vi "Autonomous Independent.vi"() -> ()   [LabVIEW 2016]
doc: "This VI is called when autonomous begins, and will automatically be terminated when autonomous ends. You can carry out timed or sensor driven robot movement independently without needing to return to the caller."
uses:
  <vilib>/Rock Robotics/WPI/DriverStation/WPI_DriverStationAllianceInfo.ctl
  Controls/Auto Selector.ctl
  Controls/Auto 1.ctl
  Controls/Auto 2.ctl
  Controls/Control 1.ctl
  Robot Global Data.vi
  <vilib>/Rock Robotics/Network Tables/NT Read Number.vi
panel:
  in  "4th distance C":dbl=2.0 format="%#_13g"
  in  "2nd Turn":dbl=49.0
  in  "3rd distance C":dbl=-0.5
  in  "2nd distance C":dbl=0.6 format="%#_13g"
  in  "1st turn C":dbl=-49.0
  in  "1st distance C":dbl=1.7
  in  "Turret angle Blue":dbl=13.0
  in  "CORRECAO":dbl=0.02
  in  "2nd distance B":dbl=0.3 format="%#_13g"
  in  "1st distance B":dbl=1.5 format="%#_13g"
  out "Red alliance?":bool
  in  "Turret angle Red":dbl=-12.0
  in  "3rd distance":dbl=-0.3 format="%#_13g"
  in  "2nd distance":dbl=0.6 format="%#_13g"
  in  "1st turn":dbl=-49.0 format="%.2f"
  in  "1st distance":dbl=1.7 format="%#_13g"
  # "vermelho = -12"
  # "azul = -13"
  # "Gear + Fuel"
  # "Gear on Feeder peg"
  # "Middle Gear"
  # "da pra reduzir  a velocidade segunda distancia"
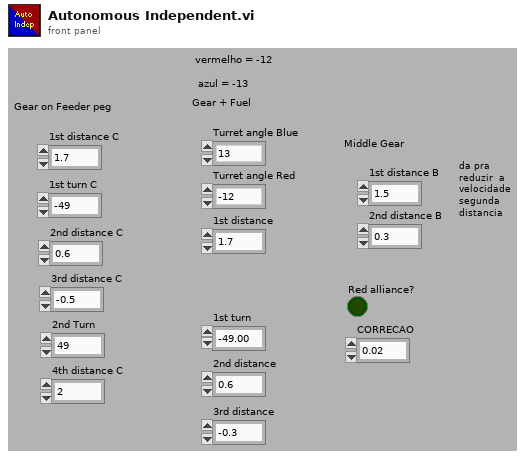
[diagram p1: front panel]
types:
  T1 = typedef "WPI_DriverStationAllianceInfo.ctl" = enum16{"Red", "Blue", "Invalid"}
  T2 = typedef "WPI_EncoderDevRef.ctl" = cluster{"DevStatus":errorcluster, "EncoderIndex":T3, "CounterIndex":T4, "DistancePerCount":dbl, "Decoding Type":T5}
  T3 = typedef "FPGA_EncoderIdx.ctl" = enum8{"Enc 0", "Enc 1", "Enc 2", "Enc 3", "Enc 4", "Enc 5", "Enc 6", "Enc 7", "Invalid"}
  T4 = typedef "FPGA_CounterCtrSystemIndex.ctl" = enum8{"Ctr 0", "Ctr 1", "Ctr 2", "Ctr 3", "Ctr 4", "Ctr 5", "Ctr 6", "Ctr 7", "Invalid"}
  T5 = typedef "WPI_EncoderType.ctl" = enum16{"1x", "2x", "4x"}
  T6 = cluster{"Yaw":dbl, "Roll":dbl, "Pitch":dbl, "Heading":dbl, "Fused Heading":dbl}
  T7 = typedef "Auto Selector.ctl" = enum16{"Gear + Fuel with Vision", "Gear + Fuel no Vision", "Middle Gear", "Gear - Feeder peg", "Nothing"}
  T8 = typedef "Auto 1.ctl" = enum16{"Prepare", "Go Forward 1", "Wait 1", "Turn Left", "Wait 2", "Go Forward 2", "Open Gear Manipulator", "Go Back", "Wait 3"}
  T9 = typedef "Auto 2.ctl" = enum16{"Prepare", "Forward", "Open", "Go Back"}
  T10 = typedef "Control 1.ctl" = enum16{"Prepare", "Go Forward 1", "Wait 1", "Turn 1", "Wait 2", "Go Forward 2", "Drop Gear", "Wait 3", "Go Back", "Wait 4", "Turn 2", "Go forward"}
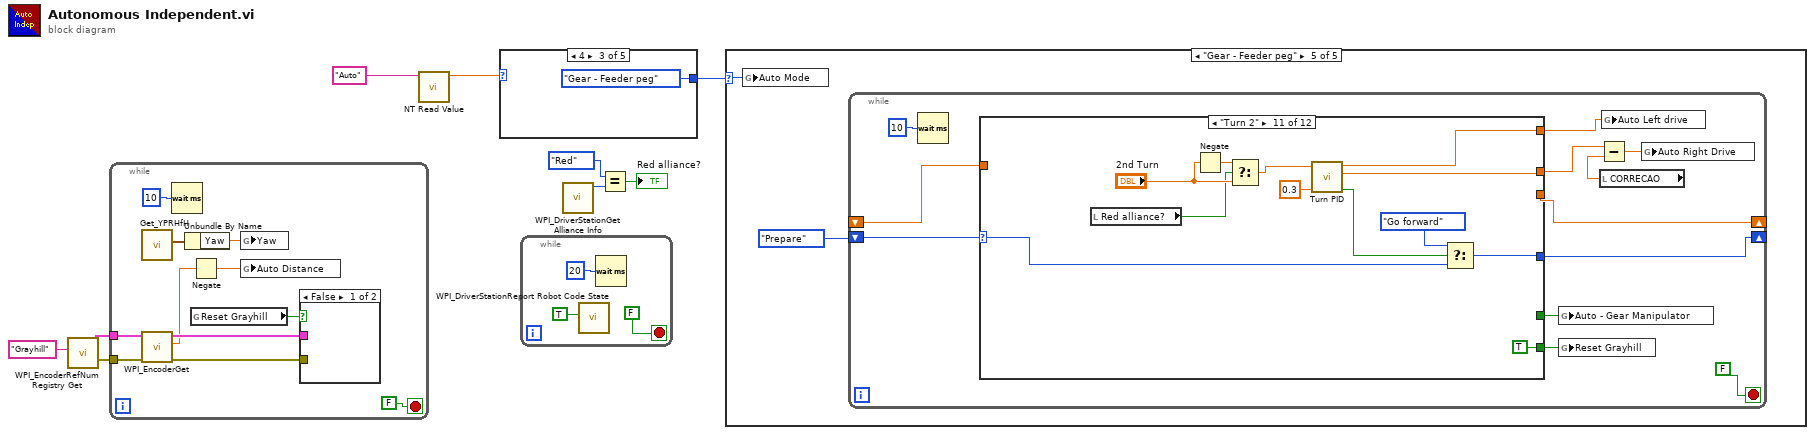
[diagram p0: block diagram]
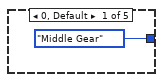
[diagram p2: hidden frame]
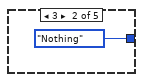
[diagram p3: hidden frame]
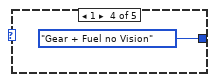
[diagram p4: hidden frame]
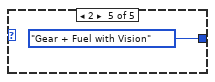
[diagram p5: hidden frame]
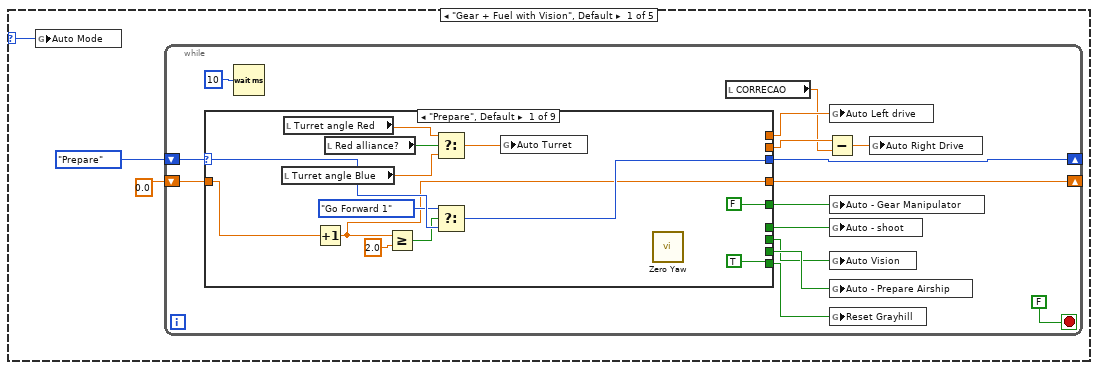
[diagram p6: hidden frame]
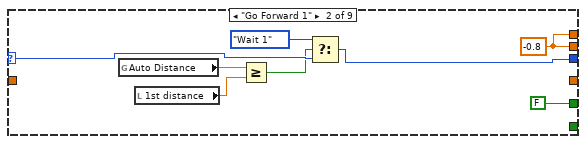
[diagram p7: hidden frame]
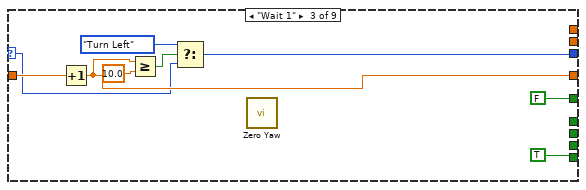
[diagram p8: hidden frame]
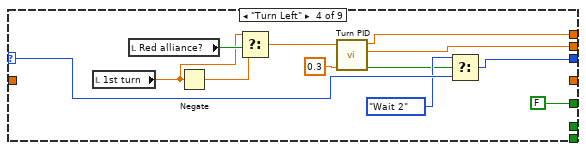
[diagram p9: hidden frame]
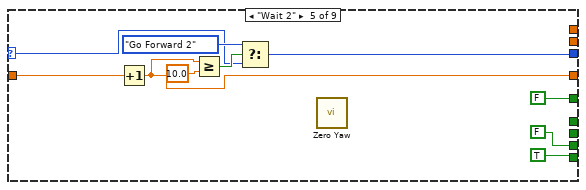
[diagram p10: hidden frame]
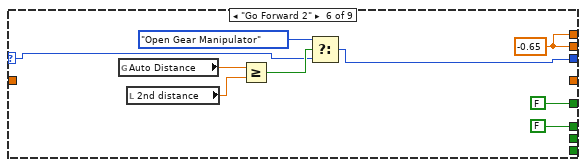
[diagram p11: hidden frame]
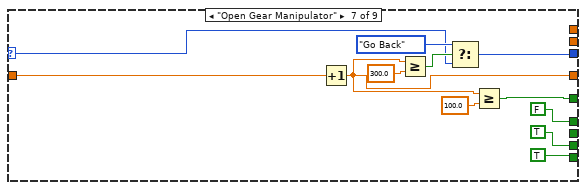
[diagram p12: hidden frame]
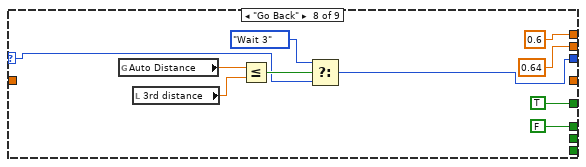
[diagram p13: hidden frame]
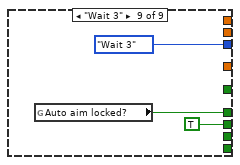
[diagram p14: hidden frame]
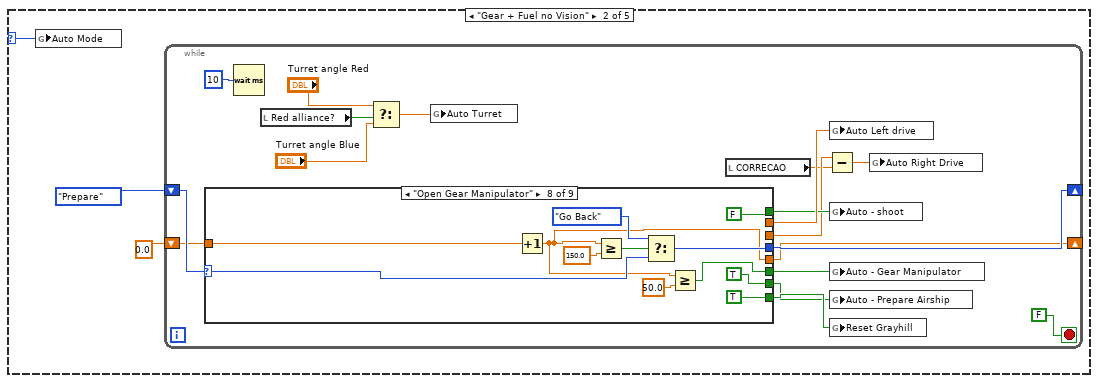
[diagram p15: hidden frame]
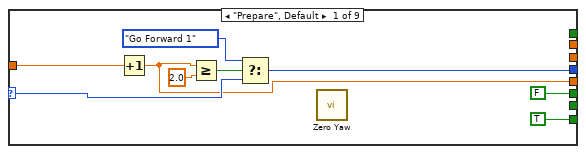
[diagram p16: hidden frame]
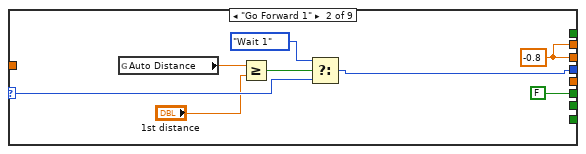
[diagram p17: hidden frame]
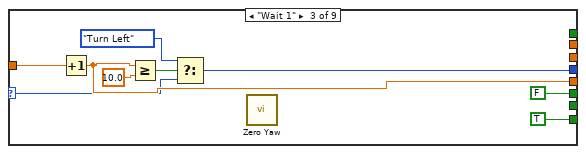
[diagram p18: hidden frame]
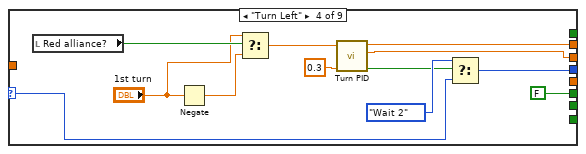
[diagram p19: hidden frame]
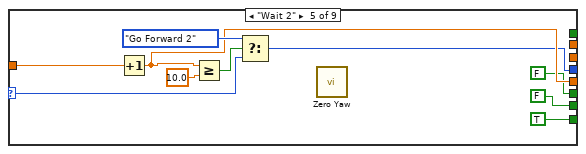
[diagram p20: hidden frame]
diagram:
  n1 = call <vilib>:"WPI_EncoderRefNum Registry Get.vi"("refnum name"="Grayhill") -> ("error out"=w7:errorcluster, "EncoderDevRef"=w8:T2)  [unwired: 9 in]
  n2 = while {
    tunnel: w8 -> [w20]
    tunnel: w7 -> [w19]
    stop <- FALSE stop-if-true
    n3 = call <vilib>:"Get_YPRHfH.vi"() -> ("YRPHfH"=w13:T6)  [unwired: 11 in]
    n4 = call <vilib>:"WPI_EncoderGet.vi"("error in (no error)"=w19, "EncoderDevRef"=w20) -> ("error out"=w17:errorcluster, "Distance"=w11:dbl, "EncoderDevRef"=w18:T2)  [unwired: 4 in, 3 out]
    n5 = Wait (ms)(milliseconds to wait=u32 10) -> ()  [unwired: 1 out]
    n6 = Unbundle By Name(w13) -> ("Yaw"=w12:dbl)
    n7 = Negate(x=w11) -> (-x=w10:dbl)
    n8 = global read "Robot Global Data.vi" "Reset Grayhill"() -> (w16:bool)
    n9 = global write "Robot Global Data.vi" "Yaw"(w12) -> ()
    n10 = global write "Robot Global Data.vi" "Auto Distance"(w10) -> ()
    n11 = case shown="False" w16 {
      tunnel: w18 -> [_ w22]
      tunnel: w17 -> [_ w21]
      frame False {
      }
      frame True {
        n12 = call <vilib>:"WPI_EncoderReset.vi"("error in (no error)"=w21, "EncoderDevRef"=w22) -> ()  [unwired: 8 in, 2 out]
      }
    }
  }
  n13 = call-poly <vilib>:"NT Read Value.vi"("Name"="Auto") -> ("Numeric"=w1:dbl)  [unwired: 9 in, 1 out]
  n14 = case shown="4" w1 {
    tunnel: [Auto_Selector."Middle Gear" Auto_Selector."Nothing" Auto_Selector."Gear - Feeder peg" Auto_Selector."Gear + Fuel no Vision" Auto_Selector."Gear + Fuel with Vision"] -> w3
    frame 0, Default {
    }
    frame 3 {
    }
    frame 4 {
    }
    frame 1 {
    }
    frame 2 {
    }
  }
  n15 = while {
    stop <- FALSE stop-if-true
    n16 = call <vilib>:"WPI_DriverStationReport Robot Code State.vi"("Autonomous"=TRUE) -> ()  [unwired: 10 in, 1 out]
    n17 = Wait (ms)(milliseconds to wait=u32 20) -> ()  [unwired: 1 out]
  }
  n18 = call <vilib>:"WPI_DriverStationGet Alliance Info.vi"() -> ("Alliance"=w6:T1)  [unwired: 11 out]
  n19 = Equal?(x=WPI_DriverStationAllianceInfo."Red" ("Alliance"), y=w6) -> (x = y?=→"Red alliance?":bool)
  n20 = case shown="\"Gear - Feeder peg\"" w3 {
    selector: w3 -> [w31 w135 w237 _ w286]
    frame "Gear + Fuel with Vision", Default {
      n21 = global write "Robot Global Data.vi" "Auto Mode"(w31) -> ()
      n22 = while {
        shift-right: [w46] -> _
        shift-left: Auto_1."Prepare" -> [w47]
        shift-right: [w44] -> _
        shift-left: 0.0 -> [w45]
        stop <- FALSE stop-if-true
        n23 = case shown="\"Prepare\", Default" w47 {
          selector: w47 -> [w60 w67 w74 w86 w94 w106 w115 w126 _]
          tunnel: [w61 w68 w75 w87 w95 w105 w118 w127 Auto_1."Wait 3"] -> w46
          tunnel: w45 -> [w58 _ w78 _ w97 _ w119 _ _]
          tunnel: [w57 _ w77 _ w96 _ w113 _ _] -> w44
          tunnel: [TRUE ("Reset Grayhill") _ TRUE ("Reset Grayhill") _ TRUE ("Reset Grayhill") _ TRUE ("Reset Grayhill") _ _] -> w42
          tunnel: [_ w69 _ w89 _ w104 _ 0.64 ("Right Out") _] -> w36
          tunnel: [_ w69 _ w88 _ w104 _ 0.6 _] -> w41
          tunnel: [FALSE ("Reset Grayhill") FALSE ("Reset Grayhill") FALSE ("Reset Grayhill") FALSE ("Reset Grayhill") FALSE ("Reset Grayhill") FALSE ("Reset Grayhill") w111 TRUE ("Reset Grayhill") _] -> w40
          tunnel: [_ _ _ _ _ FALSE FALSE FALSE w132] -> w39
          tunnel: [_ _ _ _ FALSE ("Reset Grayhill") _ TRUE ("Reset Grayhill") _ _] -> w38
          tunnel: [_ _ _ _ _ _ _ _ TRUE] -> w37
          frame "Prepare", Default {
            n24 = local read "Turret angle Blue"() -> (w49:dbl)
            n25 = local read "Turret angle Red"() -> (w50:dbl)
            n26 = Increment(x=w58) -> (x+1=w57:dbl)
            n27 = local read "Red alliance?"() -> (w51:bool)
            n28 = Greater Or Equal?(x=w57, y=2.0) -> (x >= y?=w55:bool)
            n29 = Select(t=w50, s=w51, f=w49) -> (s? t:f=w52:dbl)
            n30 = Select(t=Auto_1."Go Forward 1", s=w55, f=w60) -> (s? t:f=w61:T8)
            n31 = global write "Robot Global Data.vi" "Auto Turret"(w52) -> ()
            n32 = call <vilib>:"Zero Yaw.vi"() -> ()  [unwired: 12 in]
          }
          frame "Go Forward 1" {
            w69 = -0.8
            n33 = global read "Robot Global Data.vi" "Auto Distance"() -> (w65:dbl)
            n34 = local read "1st distance"() -> (w62:dbl)
            n35 = Greater Or Equal?(x=w65, y=w62) -> (x >= y?=w64:bool)
            n36 = Select(t=Auto_1."Wait 1", s=w64, f=w67) -> (s? t:f=w68:T8)
          }
          frame "Wait 1" {
            n37 = Increment(x=w78) -> (x+1=w77:dbl)
            n38 = Greater Or Equal?(x=w77, y=10.0) -> (x >= y?=w73:bool)
            n39 = Select(t=Auto_1."Turn Left", s=w73, f=w74) -> (s? t:f=w75:T8)
            n40 = call <vilib>:"Zero Yaw.vi"() -> ()  [unwired: 12 in]
          }
          frame "Turn Left" {
            n41 = local read "1st turn"() -> (w79:dbl)
            n42 = local read "Red alliance?"() -> (w80:bool)
            n43 = Negate(x=w79) -> (-x=w81:dbl)
            n44 = Select(t=w79, s=w80, f=w81) -> (s? t:f=w82:dbl)
            n45 = call "Turn PID.vi"("Range"=0.3, "setpoint"=w82) -> ("in range?"=w84:bool, "Right Out"=w89:dbl, "Left Out"=w88:dbl)  [unwired: 7 in]
            n46 = Select(t=Auto_1."Wait 2", s=w84, f=w86) -> (s? t:f=w87:T8)
          }
          frame "Wait 2" {
            n47 = Increment(x=w97) -> (x+1=w96:dbl)
            n48 = Greater Or Equal?(x=w96, y=10.0) -> (x >= y?=w99:bool)
            n49 = Select(t=Auto_1."Go Forward 2", s=w99, f=w94) -> (s? t:f=w95:T8)
            n50 = call <vilib>:"Zero Yaw.vi"() -> ()  [unwired: 12 in]
          }
          frame "Go Forward 2" {
            w104 = -0.65 ("Right Out")
            n51 = global read "Robot Global Data.vi" "Auto Distance"() -> (w108:dbl)
            n52 = local read "2nd distance"() -> (w101:dbl)
            n53 = Greater Or Equal?(x=w108, y=w101) -> (x >= y?=w107:bool)
            n54 = Select(t=Auto_1."Open Gear Manipulator", s=w107, f=w106) -> (s? t:f=w105:T8)
          }
          frame "Open Gear Manipulator" {
            n55 = Increment(x=w119) -> (x+1=w113:dbl)
            n56 = Greater Or Equal?(x=w113, y=300.0) -> (x >= y?=w117:bool)
            n57 = Select(t=Auto_1."Go Back", s=w117, f=w115) -> (s? t:f=w118:T8)
            n58 = Greater Or Equal?(x=w113, y=100.0) -> (x >= y?=w111:bool)
          }
          frame "Go Back" {
            n59 = global read "Robot Global Data.vi" "Auto Distance"() -> (w129:dbl)
            n60 = local read "3rd distance"() -> (w123:dbl)
            n61 = Less Or Equal?(x=w129, y=w123) -> (x <= y?=w128:bool)
            n62 = Select(t=Auto_1."Wait 3", s=w128, f=w126) -> (s? t:f=w127:T8)
          }
          frame "Wait 3" {
            n63 = global read "Robot Global Data.vi" "Auto aim locked?"() -> (w132:bool)
          }
        }
        n64 = Wait (ms)(milliseconds to wait=u32 10) -> ()  [unwired: 1 out]
        n65 = local read "CORRECAO"() -> (w34:dbl)
        n66 = Subtract(x=w36, y=w34) -> (x-y=w35:dbl)
        n67 = global write "Robot Global Data.vi" "Auto Left drive"(w41) -> ()
        n68 = global write "Robot Global Data.vi" "Auto - Gear Manipulator"(w40) -> ()
        n69 = global write "Robot Global Data.vi" "Auto - shoot"(w39) -> ()
        n70 = global write "Robot Global Data.vi" "Auto Vision"(w37) -> ()
        n71 = global write "Robot Global Data.vi" "Auto - Prepare Airship"(w38) -> ()
        n72 = global write "Robot Global Data.vi" "Reset Grayhill"(w42) -> ()
        n73 = global write "Robot Global Data.vi" "Auto Right Drive"(w35) -> ()
      }
    }
    frame "Gear + Fuel no Vision" {
      n74 = global write "Robot Global Data.vi" "Auto Mode"(w135) -> ()
      n75 = while {
        shift-right: [w153] -> _
        shift-left: Auto_1."Prepare" -> [w154]
        shift-right: [w151] -> _
        shift-left: 0.0 -> [w152]
        stop <- FALSE stop-if-true
        n76 = case shown="\"Open Gear Manipulator\"" w154 {
          selector: w154 -> [w163 w170 w177 w189 w197 _ w209 w221 w232]
          tunnel: [w164 w171 w178 w190 w198 Auto_1."Wait 3" w210 w224 w231] -> w153
          tunnel: w152 -> [w161 _ w181 _ w200 _ _ w225 _]
          tunnel: [w160 _ w180 _ w199 _ _ w219 _] -> w151
          tunnel: [TRUE ("Reset Grayhill") _ TRUE ("Reset Grayhill") _ TRUE ("Reset Grayhill") _ _ TRUE ("Reset Grayhill") _] -> w149
          tunnel: [_ w172 _ w192 _ _ 0.64 ("Right Out") _ w230] -> w141
          tunnel: [_ w172 _ w191 _ _ 0.6 _ w230] -> w148
          tunnel: [FALSE ("Reset Grayhill") FALSE ("Reset Grayhill") FALSE ("Reset Grayhill") FALSE ("Reset Grayhill") FALSE ("Reset Grayhill") _ TRUE ("Reset Grayhill") w217 FALSE ("Reset Grayhill")] -> w147
          tunnel: [_ _ _ _ _ TRUE FALSE FALSE FALSE] -> w146
          tunnel: [_ _ _ _ FALSE ("Reset Grayhill") _ _ TRUE ("Reset Grayhill") _] -> w145
          frame "Prepare", Default {
            n77 = Increment(x=w161) -> (x+1=w160:dbl)
            n78 = Greater Or Equal?(x=w160, y=2.0) -> (x >= y?=w158:bool)
            n79 = Select(t=Auto_1."Go Forward 1", s=w158, f=w163) -> (s? t:f=w164:T8)
            n80 = call <vilib>:"Zero Yaw.vi"() -> ()  [unwired: 12 in]
          }
          frame "Go Forward 1" {
            w172 = -0.8
            n81 = global read "Robot Global Data.vi" "Auto Distance"() -> (w168:dbl)
            n82 = Greater Or Equal?(x=w168, y="1st distance") -> (x >= y?=w166:bool)
            n83 = Select(t=Auto_1."Wait 1", s=w166, f=w170) -> (s? t:f=w171:T8)
          }
          frame "Wait 1" {
            n84 = Increment(x=w181) -> (x+1=w180:dbl)
            n85 = Greater Or Equal?(x=w180, y=10.0) -> (x >= y?=w176:bool)
            n86 = Select(t=Auto_1."Turn Left", s=w176, f=w177) -> (s? t:f=w178:T8)
            n87 = call <vilib>:"Zero Yaw.vi"() -> ()  [unwired: 12 in]
          }
          frame "Turn Left" {
            n88 = local read "Red alliance?"() -> (w183:bool)
            n89 = Negate(x="1st turn") -> (-x=w184:dbl)
            n90 = Select(t="1st turn", s=w183, f=w184) -> (s? t:f=w185:dbl)
            n91 = call "Turn PID.vi"("Range"=0.3, "setpoint"=w185) -> ("in range?"=w187:bool, "Right Out"=w192:dbl, "Left Out"=w191:dbl)  [unwired: 7 in]
            n92 = Select(t=Auto_1."Wait 2", s=w187, f=w189) -> (s? t:f=w190:T8)
          }
          frame "Wait 2" {
            n93 = Increment(x=w200) -> (x+1=w199:dbl)
            n94 = Greater Or Equal?(x=w199, y=10.0) -> (x >= y?=w202:bool)
            n95 = Select(t=Auto_1."Go Forward 2", s=w202, f=w197) -> (s? t:f=w198:T8)
            n96 = call <vilib>:"Zero Yaw.vi"() -> ()  [unwired: 12 in]
          }
          frame "Wait 3" {
          }
          frame "Go Back" {
            n97 = global read "Robot Global Data.vi" "Auto Distance"() -> (w213:dbl)
            n98 = Less Or Equal?(x=w213, y="3rd distance") -> (x <= y?=w211:bool)
            n99 = Select(t=Auto_1."Wait 3", s=w211, f=w209) -> (s? t:f=w210:T8)
          }
          frame "Open Gear Manipulator" {
            n100 = Increment(x=w225) -> (x+1=w219:dbl)
            n101 = Greater Or Equal?(x=w219, y=150.0) -> (x >= y?=w223:bool)
            n102 = Select(t=Auto_1."Go Back", s=w223, f=w221) -> (s? t:f=w224:T8)
            n103 = Greater Or Equal?(x=w219, y=50.0) -> (x >= y?=w217:bool)
          }
          frame "Go Forward 2" {
            w230 = -0.65 ("Right Out")
            n104 = global read "Robot Global Data.vi" "Auto Distance"() -> (w235:dbl)
            n105 = Greater Or Equal?(x=w235, y="2nd distance") -> (x >= y?=w233:bool)
            n106 = Select(t=Auto_1."Open Gear Manipulator", s=w233, f=w232) -> (s? t:f=w231:T8)
          }
        }
        n107 = Wait (ms)(milliseconds to wait=u32 10) -> ()  [unwired: 1 out]
        n108 = local read "Red alliance?"() -> (w143:bool)
        n109 = Select(t="Turret angle Red", s=w143, f="Turret angle Blue") -> (s? t:f=w142:dbl)
        n110 = global write "Robot Global Data.vi" "Auto Turret"(w142) -> ()
        n111 = local read "CORRECAO"() -> (w139:dbl)
        n112 = Subtract(x=w141, y=w139) -> (x-y=w140:dbl)
        n113 = global write "Robot Global Data.vi" "Auto Left drive"(w148) -> ()
        n114 = global write "Robot Global Data.vi" "Auto - shoot"(w146) -> ()
        n115 = global write "Robot Global Data.vi" "Auto - Gear Manipulator"(w147) -> ()
        n116 = global write "Robot Global Data.vi" "Auto - Prepare Airship"(w145) -> ()
        n117 = global write "Robot Global Data.vi" "Reset Grayhill"(w149) -> ()
        n118 = global write "Robot Global Data.vi" "Auto Right Drive"(w140) -> ()
      }
    }
    frame "Middle Gear" {
      n119 = global write "Robot Global Data.vi" "Auto Mode"(w237) -> ()
      n120 = while {
        shift-right: [w243] -> _
        shift-left: Auto_2."Prepare" -> [w250]
        shift-right: [w246] -> _
        shift-left: _ -> [w247]
        stop <- FALSE stop-if-true
        n121 = case shown="\"Forward\"" w250 {
          selector: w250 -> [w253 w267 w270 _]
          tunnel: [TRUE _ _ _] -> w249
          tunnel: [FALSE _ w269 TRUE] -> w248
          tunnel: w247 -> [w258 _ w273 _]
          tunnel: [w257 _ w272 _] -> w246
          tunnel: [w255 w261 _ w282] -> w241
          tunnel: [w255 w261 _ w282] -> w244
          tunnel: [w252 w266 w271 Auto_2."Go Back"] -> w243
          frame "Prepare", Default {
            w255 = 0.0
            n122 = Increment(x=w258) -> (x+1=w257:dbl)
            n123 = Greater Or Equal?(x=w257, y=5.0) -> (x >= y?=w254:bool)
            n124 = Select(t=Auto_2."Forward", s=w254, f=w253) -> (s? t:f=w252:T9)
          }
          frame "Forward" {
            w261 = -0.8
            n125 = global read "Robot Global Data.vi" "Auto Distance"() -> (w265:dbl)
            n126 = Greater Or Equal?(x=w265, y="1st distance B") -> (x >= y?=w263:bool)
            n127 = Select(t=Auto_2."Open", s=w263, f=w267) -> (s? t:f=w266:T9)
          }
          frame "Open" {
            n128 = Increment(x=w273) -> (x+1=w272:dbl)
            n129 = Greater Or Equal?(x=w272, y=200.0) -> (x >= y?=w275:bool)
            n130 = Select(t=Auto_2."Go Back", s=w275, f=w270) -> (s? t:f=w271:T9)
            n131 = Greater Or Equal?(x=w272, y=50.0) -> (x >= y?=w269:bool)
          }
          frame "Go Back" {
            n132 = global read "Robot Global Data.vi" "Auto Distance"() -> (w280:dbl)
            n133 = Less Or Equal?(x=w280, y="2nd distance B") -> (x <= y?=w278:bool)
            n134 = case shown="False" w278 {
              tunnel: [0.6 0.0] -> w282
              frame False {
              }
              frame True {
              }
            }
          }
        }
        n135 = Wait (ms)(milliseconds to wait=u32 10) -> ()  [unwired: 1 out]
        n136 = global write "Robot Global Data.vi" "Auto Left drive"(w244) -> ()
        n137 = global write "Robot Global Data.vi" "Auto - Gear Manipulator"(w248) -> ()
        n138 = global write "Robot Global Data.vi" "Reset Grayhill"(w249) -> ()
        n139 = Subtract(x=w241, y="CORRECAO") -> (x-y=w239:dbl)
        n140 = global write "Robot Global Data.vi" "Auto Right Drive"(w239) -> ()
      }
    }
    frame "Nothing" {
    }
    frame "Gear - Feeder peg" {
      n141 = global write "Robot Global Data.vi" "Auto Mode"(w286) -> ()
      n142 = while {
        shift-right: [w292] -> _
        shift-left: Control_1."Prepare" -> [w296]
        shift-right: [w293] -> _
        shift-left: _ -> [w294]
        stop <- FALSE stop-if-true
        n143 = Wait (ms)(milliseconds to wait=u32 10) -> ()  [unwired: 1 out]
        n144 = case shown="\"Turn 2\"" w296 {
          selector: w296 -> [w302 w309 w316 w324 w336 w344 w351 w361 w368 w375 w383 _]
          tunnel: [TRUE _ TRUE _ TRUE _ TRUE TRUE _ _ TRUE _] -> w295
          tunnel: w294 -> [w304 _ w321 _ w339 _ w354 w364 _ w378 _ _]
          tunnel: [w305 _ w320 _ w340 _ w356 w365 _ w379 _ _] -> w293
          tunnel: [w301 w310 w317 w325 w337 w345 w349 w362 w369 w373 w385 Control_1."Go forward"] -> w292
          tunnel: [_ w313 _ w326 _ w341 _ _ w372 _ w386 w395] -> w289
          tunnel: [_ w313 _ w327 _ w341 _ _ w372 _ w387 w395] -> w288
          tunnel: [_ _ _ _ _ _ w352 _ _ _ _ _] -> w287
          frame "Prepare", Default {
            n145 = Greater?(x=w304, y=2.0) -> (0:w299:bool)
            n146 = Increment(x=w304) -> (x+1=w305:dbl)
            n147 = Select(t=Control_1."Go Forward 1", s=w299, f=w302) -> (s? t:f=w301:T10)
            n148 = call <vilib>:"Zero Yaw.vi"() -> ()  [unwired: 12 in]
          }
          frame "Go Forward 1" {
            w313 = -0.8
            n149 = global read "Robot Global Data.vi" "Auto Distance"() -> (w312:dbl)
            n150 = Greater Or Equal?(x=w312, y="1st distance C") -> (x >= y?=w308:bool)
            n151 = Select(t=Control_1."Wait 1", s=w308, f=w309) -> (s? t:f=w310:T10)
          }
          frame "Wait 1" {
            n152 = call <vilib>:"Zero Yaw.vi"() -> ()  [unwired: 12 in]
            n153 = Greater Or Equal?(x=w321, y=10.0) -> (x >= y?=w315:bool)
            n154 = Increment(x=w321) -> (x+1=w320:dbl)
            n155 = Select(t=Control_1."Turn 1", s=w315, f=w316) -> (s? t:f=w317:T10)
          }
          frame "Turn 1" {
            n156 = local read "Red alliance?"() -> (w330:bool)
            n157 = Negate(x="1st turn C") -> (-x=w328:dbl)
            n158 = Select(t=w328, s=w330, f="1st turn C") -> (s? t:f=w331:dbl)
            n159 = call "Turn PID.vi"("Range"=0.3, "setpoint"=w331) -> ("in range?"=w323:bool, "Right Out"=w326:dbl, "Left Out"=w327:dbl)  [unwired: 7 in]
            n160 = Select(t=Control_1."Wait 2", s=w323, f=w324) -> (s? t:f=w325:T10)
          }
          frame "Wait 2" {
            n161 = Greater Or Equal?(x=w339, y=10.0) -> (x >= y?=w335:bool)
            n162 = Increment(x=w339) -> (x+1=w340:dbl)
            n163 = Select(t=Control_1."Go Forward 2", s=w335, f=w336) -> (s? t:f=w337:T10)
          }
          frame "Go Forward 2" {
            w341 = -0.65
            n164 = global read "Robot Global Data.vi" "Auto Distance"() -> (w347:dbl)
            n165 = Greater Or Equal?(x=w347, y="2nd distance C") -> (x >= y?=w343:bool)
            n166 = Select(t=Control_1."Drop Gear", s=w343, f=w344) -> (s? t:f=w345:T10)
          }
          frame "Drop Gear" {
            n167 = Greater Or Equal?(x=w354, y=50.0) -> (x >= y?=w352:bool)
            n168 = Greater Or Equal?(x=w354, y=150.0) -> (x >= y?=w350:bool)
            n169 = Select(t=Control_1."Wait 3", s=w350, f=w351) -> (s? t:f=w349:T10)
            n170 = Increment(x=w354) -> (x+1=w356:dbl)
          }
          frame "Wait 3" {
            n171 = call <vilib>:"Zero Yaw.vi"() -> ()  [unwired: 12 in]
            n172 = Greater Or Equal?(x=w364, y=10.0) -> (x >= y?=w360:bool)
            n173 = Increment(x=w364) -> (x+1=w365:dbl)
            n174 = Select(t=Control_1."Go Back", s=w360, f=w361) -> (s? t:f=w362:T10)
          }
          frame "Go Back" {
            w372 = 0.65
            n175 = global read "Robot Global Data.vi" "Auto Distance"() -> (w371:dbl)
            n176 = Less Or Equal?(x=w371, y="3rd distance C") -> (x <= y?=w367:bool)
            n177 = Select(t=Control_1."Wait 4", s=w367, f=w368) -> (s? t:f=w369:T10)
          }
          frame "Wait 4" {
            n178 = Greater Or Equal?(x=w378, y=10.0) -> (x >= y?=w376:bool)
            n179 = Select(t=Control_1."Turn 2", s=w376, f=w375) -> (s? t:f=w373:T10)
            n180 = Increment(x=w378) -> (x+1=w379:dbl)
          }
          frame "Turn 2" {
            n181 = local read "Red alliance?"() -> (w380:bool)
            n182 = Negate(x="2nd Turn") -> (-x=w389:dbl)
            n183 = Select(t=w389, s=w380, f="2nd Turn") -> (s? t:f=w390:dbl)
            n184 = call "Turn PID.vi"("Range"=0.3, "setpoint"=w390) -> ("in range?"=w384:bool, "Right Out"=w386:dbl, "Left Out"=w387:dbl)  [unwired: 7 in]
            n185 = Select(t=Control_1."Go forward", s=w384, f=w383) -> (s? t:f=w385:T10)
          }
          frame "Go forward" {
            n186 = global read "Robot Global Data.vi" "Auto Distance"() -> (w397:dbl)
            n187 = Greater Or Equal?(x=w397, y="4th distance C") -> (x >= y?=w392:bool)
            n188 = Select(t=0.0, s=w392, f=-0.8) -> (s? t:f=w395:dbl)
          }
        }
        n189 = global write "Robot Global Data.vi" "Auto - Gear Manipulator"(w287) -> ()
        n190 = global write "Robot Global Data.vi" "Reset Grayhill"(w295) -> ()
        n191 = local read "CORRECAO"() -> (w290:dbl)
        n192 = Subtract(x=w289, y=w290) -> (x-y=w291:dbl)
        n193 = global write "Robot Global Data.vi" "Auto Left drive"(w288) -> ()
        n194 = global write "Robot Global Data.vi" "Auto Right Drive"(w291) -> ()
      }
    }
  }
